vi "TableLimits.vi"(7 "PNGs in folder":string[](array[string]), 8 "error in (no error)":errorcluster, 11 "Folder path":path) -> (0 "error out":errorcluster, 4 "Table limits":T1)   [LabVIEW 2023]
panel:
  out "Y":i32
  out "X":i32
  in  "Dark Blue Range":T2={"Rmin"=0, "Rmax"=24, " Gmin"=0, " Gmax"=49, " Bmin"=100, "Bmax"=119}
  in  "Current":T1
  in  "Initial":T1
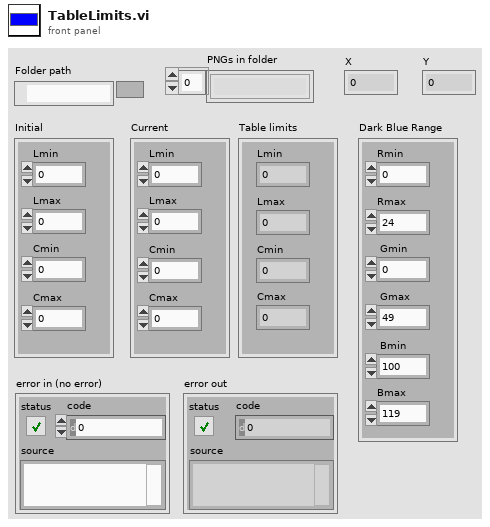
[diagram p1: front panel]
types:
  T1 = cluster{"Lmin":i32, "Lmax":i32, "Cmin":i32, "Cmax":i32}
  T2 = cluster{"Rmin":u8, "Rmax":u8, " Gmin":u8, " Gmax":u8, " Bmin":u8, "Bmax":u8}
  T3 = typedef "imagedata.ctl" = cluster{"image type":i32, "image depth":i32, "image":u8[], "mask":u8[], "colors":u32[], "Rectangle":cluster{"left":i16, "top":i16, "right":i16, "bottom":i16}}
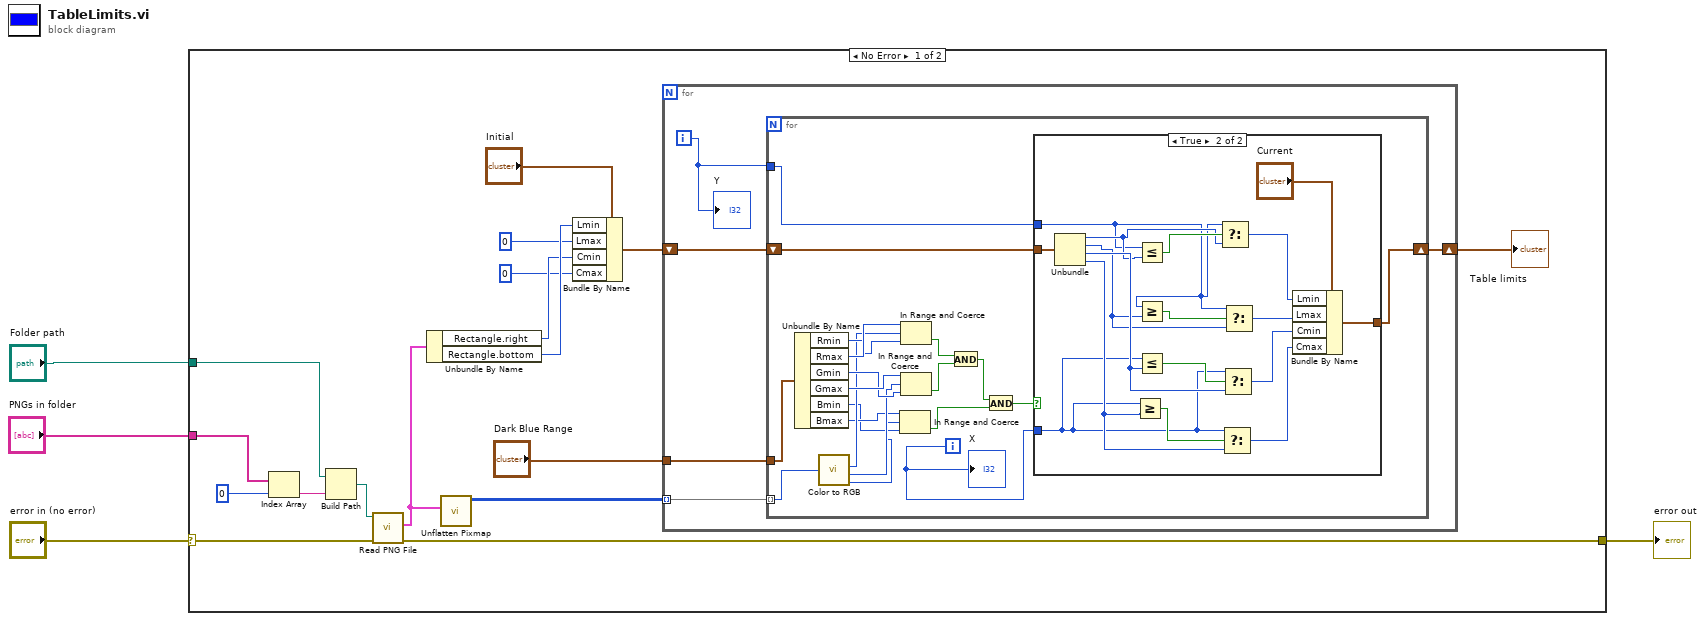
[diagram p0: block diagram]
diagram:
  n1 = case shown="No Error" "error in (no error)" {
    selector: "error in (no error)" -> [w16 w65]
    tunnel: "Folder path" -> [w19 _]
    tunnel: "PNGs in folder" -> [w20 _]
    tunnel: [w15 w65] -> w1
    frame No Error {
      n2 = Index Array(array=w20, index=0) -> (element=w18:string)
      n3 = Build Path(base path=w19, name or relative path=w18) -> (appended path=w17:path)
      n4 = call <vilib>:"Read PNG File.vi"("error in (no error)"=w16, "path to PNG file"=w17) -> ("error out"=w15:errorcluster, "image data"=w14:T3)  [unwired: 7 in, 1 out]
      n5 = Unbundle By Name(w14) -> ("Rectangle.right"=w11:i16, "Rectangle.bottom"=w12:i16)
      n6 = call <vilib>:"Unflatten Pixmap.vi"("image data"=w14) -> ("24-bit pixmap"=w7:u32[][])  [unwired: 4 in, 6 out]
      n7 = Bundle By Name(cluster="Initial", "Lmin"=w12, "Lmax"=0, "Cmin"=w11, "Cmax"=0) -> (w8:T1)
      n8 = for {
        tunnel: w7 -> [w23] mode=indexing
        tunnel: "Dark Blue Range" -> [w24]
        shift-right: [w22] -> w5
        shift-left: w8 -> [w26]
        i -> [w25]
        n9 = for {
          tunnel: w25 -> [w27]
          tunnel: w24 -> [w45]
          tunnel: w23 -> [w44] mode=indexing
          shift-right: [w28] -> w22
          shift-left: w26 -> [w46]
          i -> [w29]
          n10 = Unbundle By Name(w45) -> ("Rmin"=w42:u8, "Rmax"=w43:u8, "Gmin"=w40:u8, "Gmax"=w41:u8, "Bmin"=w36:u8, "Bmax"=w37:u8)
          n11 = call <vilib>:"Color to RGB.vi"("Color"=w44) -> ("R"=w39:u8, "G"=w38:u8, "B"=w35:u8)  [unwired: 1 out]
          n12 = In Range and Coerce(upper limit=w37, x=w35, lower limit=w36) -> (In Range?=w32:bool)  [unwired: 1 out]
          n13 = In Range and Coerce(upper limit=w43, x=w39, lower limit=w42) -> (In Range?=w34:bool)  [unwired: 1 out]
          n14 = In Range and Coerce(upper limit=w41, x=w38, lower limit=w40) -> (In Range?=w33:bool)  [unwired: 1 out]
          n15 = And(x=w34, y=w33) -> (x .and. y?=w31:bool)
          n16 = And(x=w31, y=w32) -> (x .and. y?=w30:bool)
          n17 = case shown="True" w30 {
            tunnel: w46 -> [w47 w64]
            tunnel: w29 -> [_ w51]
            tunnel: [w47 w62] -> w28
            tunnel: w27 -> [_ w48]
            frame False {
            }
            frame True {
              n18 = Unbundle(w64) -> ("Lmin"=w49:i32, "Lmax"=w50:i32, "Cmin"=w52:i32, "Cmax"=w53:i32)
              n19 = Greater Or Equal?(x=w51, y=w53) -> (x >= y?=w54:bool)
              n20 = Less Or Equal?(x=w48, y=w49) -> (x <= y?=w57:bool)
              n21 = Greater Or Equal?(x=w48, y=w50) -> (x >= y?=w56:bool)
              n22 = Less Or Equal?(x=w51, y=w52) -> (x <= y?=w55:bool)
              n23 = Select(t=w48, s=w57, f=w49) -> (s? t:f=w61:i32)
              n24 = Select(t=w51, s=w54, f=w53) -> (s? t:f=w58:i32)
              n25 = Select(t=w51, s=w55, f=w52) -> (s? t:f=w59:i32)
              n26 = Select(t=w48, s=w56, f=w50) -> (s? t:f=w60:i32)
              n27 = Bundle By Name(cluster="Current", "Lmin"=w61, "Lmax"=w60, "Cmin"=w59, "Cmax"=w58) -> (w62:T1)
            }
          }
          "X" <- w29
        }
        "Y" <- w25
      }
      "Table limits" <- w5
    }
    frame Error {
    }
  }
  "error out" <- w1
